vi "CameraControl.vi"() -> ()   [LabVIEW 2014]
uses:
  Libraries/atmcd32d.llb/ReadMode_mode typedef.ctl
  Libraries/atmcd32d.llb/AcquisitionMode_mode typedef.ctl
  Libraries/atmcd32d.llb/HSSpeed_type typedef.ctl
  Libraries/atmcd32d.llb/TriggerMode_mode typedef.ctl
  Libraries/atmcd32d.llb/Shutter_mode typedef.ctl
  Globals/AndorImage.vi
panel:
  in  "Take Video":bool
  out "Set Image Return":u32
  in  "Set Kinetic Series Number":i32=1
  in  "Set Number of Accumulations":i32=1
  in  "Set Horizontal Speed":u16(ring)=3 items=["1 MHz", "5 MHz", "10 MHz", "17 MHz"]
  out "Set Vertical Shift Speed Return":u32=20002
  in  "Set Vertical Shift Speed":u16(ring)=4 items=["0.3 us", "0.5 us", "0.9 us", "1.7 us", "3.3 us"]
  out "Vertical Shift Speed [us]":sgl format="%.1f"
  out "Set Shutter Return":u32=20002
  out "Intensity Graph":i32[][](graph)
  in  "vend":i32=512
  in  "vstart":i32=1
  in  "hend":i32=512
  in  "hstart":i32=1
  in  "vbin":i32=1
  in  "hbin":i32=1
  in  "Set Trigger":T1
  out "Return from Start Acquisition":u32=20002
  out "Return from Get Acquisition":u32=20002
  out "Exposure Time":sgl=0.01 format="%.2f"
  out "Return from GetStatus":u32=73
  in  "Take Image":bool=TRUE
  out "PreAmp Gains":i32=3
  out "EM Gain":u32
  out "Temperature [C]":i32=-70
  in  "Set EM Gain":i32
  in  "Read Settings":bool=TRUE
  in  "Stop":bool
  in  "Set Exposure Time [s]":sgl=0.01 format="%.2f"
  in  "Write Settings":bool
  in  "Set Temperature [C]":i32=-80
  out "DLL error code\n(20002 = Success)":u32=20002
  in  "Set Readout Amplifier":T2
  in  "Set Acquisition Mode":T3=enum."Kinetics"
  in  "Set Read Mode":T4=enum."Image"
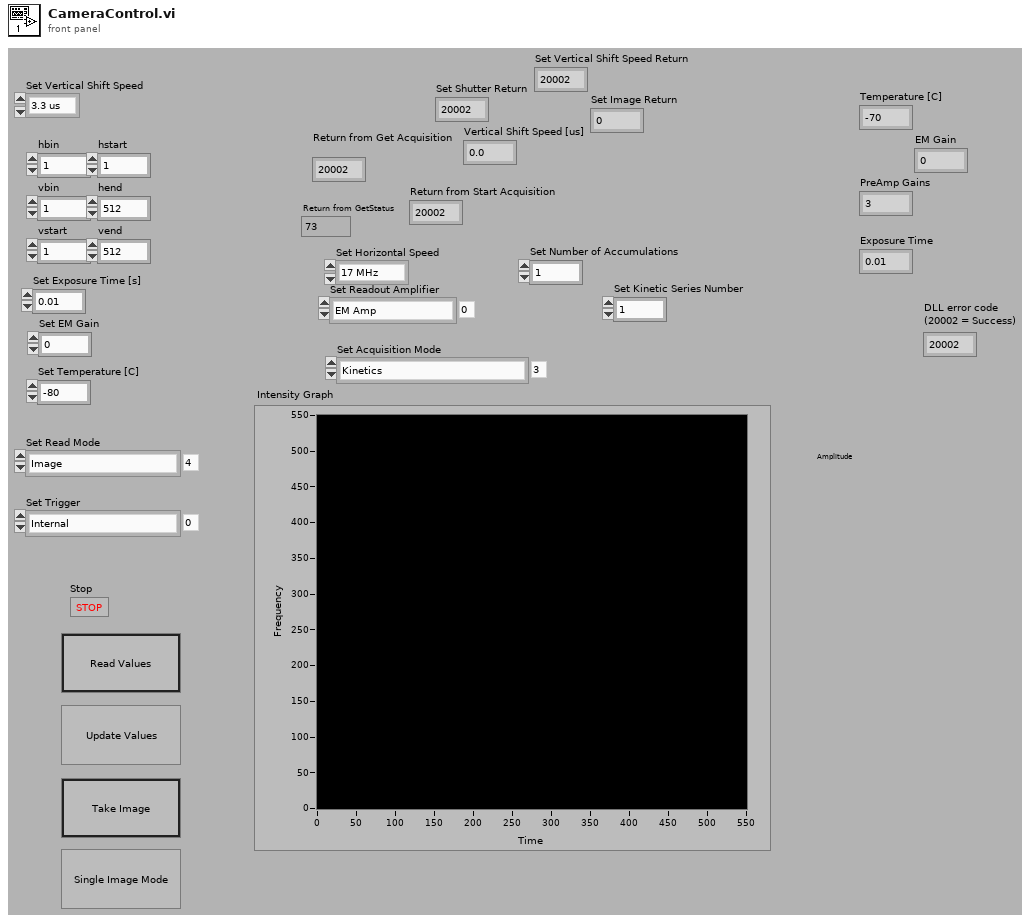
[diagram p1: front panel]
types:
  T1 = typedef "TriggerMode_mode typedef.ctl" = enum16{"Internal", "External", "N/A (2)", "N/A (3)", "N/A (4)", "N/A (5)", "External Start", "External Exposure (Bulb)", "N/A (8)", "External FVB EM", "Software", "N/A (11)", "External Charge Shifting"}
  T2 = typedef "HSSpeed_type typedef.ctl" = enum16{"EM Amp", "Conventional Amp"}
  T3 = typedef "AcquisitionMode_mode typedef.ctl" = enum16{"Reserved (0)", "Single Scan", "Accumulate", "Kinetics", "Fast Kinetics", "Run Till Abort", "Reserved (6)", "Reserved (7)", "Reserved (8)", "Time Delayed Integration"}
  T4 = typedef "ReadMode_mode typedef.ctl" = enum16{"Full Vertical Binning", "Multi-Track", "Random-Track", "Single-Track", "Image"}
  T5 = typedef "Shutter_mode typedef.ctl" = enum16{"Auto", "Open", "Close", "N/A (3)", "Open FVB Series", "Open Any Series"}
  T6 = typedef "Error Code Enum typedef.ctl" = enum32{"N/A (0)", "DRV_ERROR_CODES", "DRV_SUCCESS", "DRV_VXDNOTINSTALLED", "DRV_ERROR_SCAN", "DRV_ERROR_CHECK_SUM", "DRV_ERROR_FILELOAD", "DRV_UNKNOWN_FUNC", "DRV_ERROR_VXD_INIT", "DRV_ERROR_ADDRESS", "DRV_ERROR_PAGELOCK", "DRV_ERROR_PAGEUNLOCK", "DRV_ERROR_BOARDTEST", "DRV_ERROR_ACK", "DRV_ERROR_UP_FIFO", "DRV_ERROR_PATTERN", "N/A (16)", "DRV_ACQUISITION_ERRORS", "DRV_ACQ_BUFFER", "DRV_ACQ_DOWNFIFO_FULL", "DRV_PROC_UNKONWN_INSTRUCTION", "DRV_ILLEGAL_OP_CODE", "DRV_KINETIC_TIME_NOT_MET", "DRV_ACCUM_TIME_NOT_MET", "DRV_NO_NEW_DATA", "N/A (25)", "DRV_SPOOLERROR", "N/A (27)", "N/A (28)", "N/A (29)", "N/A (30)", "N/A (31)", "N/A (32)", "DRV_TEMPERATURE_CODES", "DRV_TEMPERATURE_OFF", "DRV_TEMPERATURE_NOT_STABILIZED", "DRV_TEMPERATURE_STABILIZED", "DRV_TEMPERATURE_NOT_REACHED", "DRV_TEMPERATURE_OUT_RANGE", "DRV_TEMPERATURE_NOT_SUPPORTED", "DRV_TEMPERATURE_DRIFT", "N/A (41)", "N/A (42)", "N/A (43)", "N/A (44)", "N/A (45)", "N/A (46)", "N/A (47)", "N/A (48)", "DRV_GENERAL_ERRORS", "DRV_INVALID_AUX", "DRV_COF_NOTLOADED", "DRV_FPGAPROG", "DRV_FLEXERROR", "DRV_GPIBERROR", "N/A (55)", "N/A (56)", "N/A (57)", "N/A (58)", "N/A (59)", "N/A (60)", "N/A (61)", "N/A (62)", "N/A (63)", "DRV_DATATYPE", "DRV_DRIVER_ERRORS", "DRV_P1INVALID", "DRV_P2INVALID", "DRV_P3INVALID", "DRV_P4INVALID", "DRV_INIERROR", "DRV_COFERROR", "DRV_ACQUIRING", "DRV_IDLE", "DRV_TEMPCYCLE", "DRV_NOT_INITIALIZED", "DRV_P5INVALID", "DRV_P6INVALID", "DRV_INVALID_MODE", "DRV_INVALID_FILTER", "DRV_I2CERRORS", "DRV_I2CDEVNOTFOUND", "DRV_I2CTIMEOUT", "DRV_P7INVALID", "N/A (84)", "N/A (85)", "N/A (86)", "N/A (87)", "N/A (88)", "N/A (89)", "DRV_IOCERROR", "DRV_VRMVERSIONERROR"}
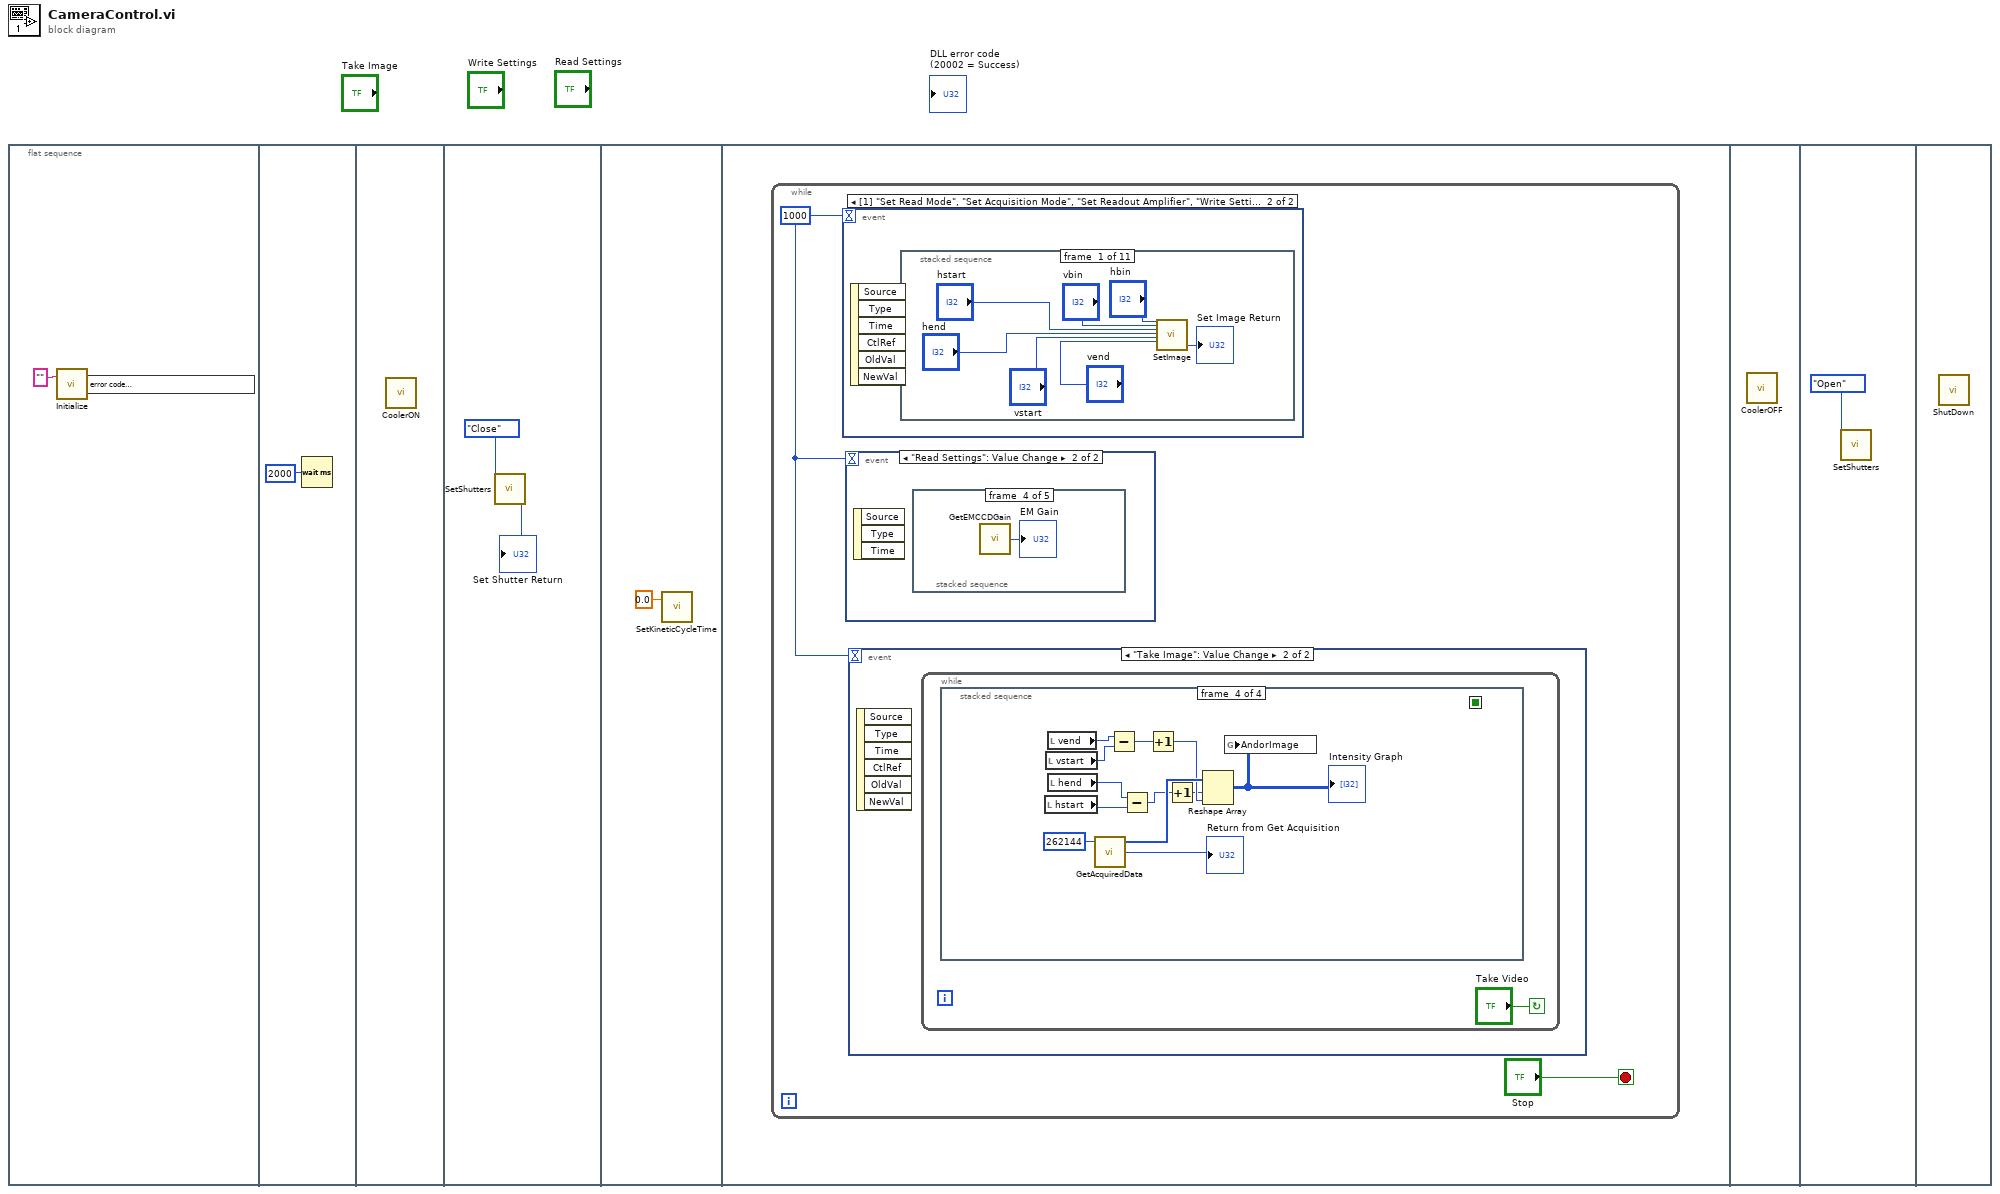
[diagram p0: block diagram]
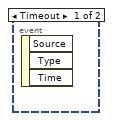
[diagram p2: hidden frame]
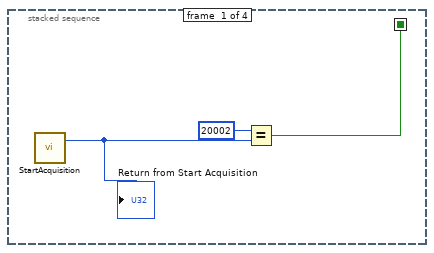
[diagram p3: hidden frame]
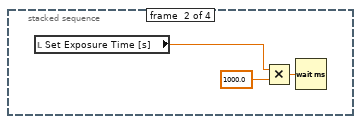
[diagram p4: hidden frame]
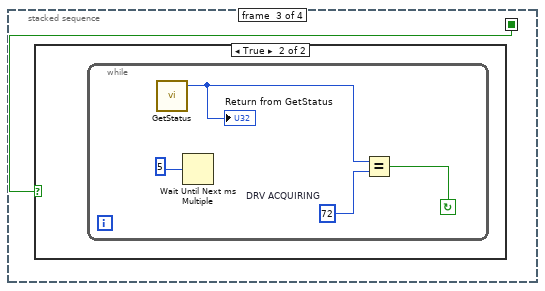
[diagram p5: hidden frame]
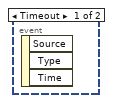
[diagram p7: hidden frame]
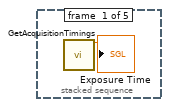
[diagram p8: hidden frame]
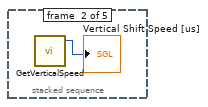
[diagram p9: hidden frame]
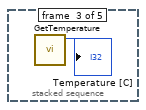
[diagram p10: hidden frame]
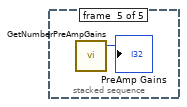
[diagram p11: hidden frame]
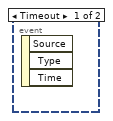
[diagram p12: hidden frame]
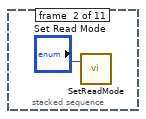
[diagram p13: hidden frame]
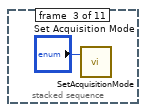
[diagram p14: hidden frame]
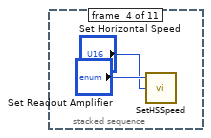
[diagram p15: hidden frame]
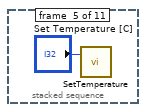
[diagram p16: hidden frame]
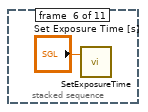
[diagram p17: hidden frame]
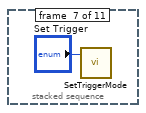
[diagram p18: hidden frame]
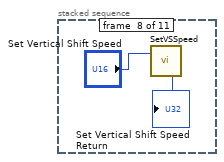
[diagram p19: hidden frame]
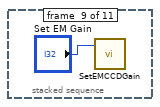
[diagram p20: hidden frame]
diagram:
  n1 = flat-sequence {
    frame #0 {
      n2 = call "Initialize.vi"("directory (\"\")"="" ("directory (\"\")")) -> ("DLL error code"=w1:u32)  [unwired: 1 in, 1 out]
      n3 = local write "DLL error code\n(20002 = Success)"(w1) -> ()
    }
    frame #1 {
      n4 = Wait (ms)(milliseconds to wait=u32 2000) -> ()  [unwired: 1 out]
    }
    frame #2 {
      n5 = call "CoolerON.vi"() -> ()  [unwired: 2 in, 2 out]
    }
    frame #3 {
      n6 = call "SetShutters.vi"("mode"=Shutter_mode_typedef."Close") -> ("DLL error code"=→"Set Shutter Return":u32)  [unwired: 17 in, 1 out]
    }
    frame #4 {
      n7 = call "SetKineticCycleTime.vi"("time"=sgl 0.0) -> ()  [unwired: 1 in, 2 out]
    }
    frame #5 {
      n8 = while {
        stop <- "Stop" stop-if-true
        w7 = 1000
        n9 = event shown="[1] \"Set Read Mode\", \"Set Acquisition Mode\", \"Set Readout Amplifier\", \"Write Settings\", \"Set Temperature [C]\", \"Set Exposure Time [s]\", \"Set Trigger\", \"hbin\", \"vbin\", \"hstart\", \"hend\", \"vstart\", \"vend\", \"Set EM Gain\", \"Set Vertical Shift Speed\", \"Set Vertical Shift Speed Return\", \"Set Horizontal Speed\", \"Set Number of Accumulations\", \"Set Kinetic Series Number\": Value Change" {
          selector: _ -> [_ _]
          dyn-events: _ -> [_ _]
          timeout: w7 -> [_ _]
          event Timeout {
            n10 = event-data() -> ()  [unwired: 1 in, 3 out]
          }
          event "Write Settings", "Set Temperature [C]", "Set Exposure Time [s]", "hbin", "vbin", "hstart", "hend", "vstart", "vend", "Set EM Gain", "Set Vertical Shift Speed", "Set Vertical Shift Speed Return", "Set Horizontal Speed", "Set Number of Accumulations", "Set Kinetic Series Number": Value Change {
            n11 = event-data() -> ()  [unwired: 1 in, 6 out]
            n12 = stacked-sequence {
              frame #0 {
                n13 = call "SetImage.vi"("hbin"="hbin", "vbin"="vbin", "hstart"="hstart", "hend"="hend", "vstart"="vstart", "vend"="vend") -> ("DLL error code"=→"Set Image Return":u32)  [unwired: 20 in, 1 out]
              }
              frame #1 {
                n14 = call "SetReadMode.vi"("mode"="Set Read Mode") -> ()  [unwired: 1 in, 2 out]
              }
              frame #2 {
                n15 = call "SetAcquisitionMode.vi"("mode"="Set Acquisition Mode") -> ()  [unwired: 1 in, 2 out]
              }
              frame #3 {
                n16 = call "SetHSSpeed.vi"("index"="Set Horizontal Speed", "type"="Set Readout Amplifier") -> ()  [unwired: 2 in, 2 out]
              }
              frame #4 {
                n17 = call "SetTemperature.vi"("temperature"="Set Temperature [C]") -> ()  [unwired: 1 in, 2 out]
              }
              frame #5 {
                n18 = call "SetExposureTime.vi"("time"="Set Exposure Time [s]") -> ()  [unwired: 1 in, 2 out]
              }
              frame #6 {
                n19 = call "SetTriggerMode.vi"("mode"="Set Trigger") -> ()  [unwired: 1 in, 2 out]
              }
              frame #7 {
                n20 = call "SetVSSpeed.vi"("index"="Set Vertical Shift Speed") -> ("DLL error code"=→"Set Vertical Shift Speed Return":u32)  [unwired: 1 in, 1 out]
              }
              frame #8 {
                n21 = call "SetEMCCDGain.vi"("gain"="Set EM Gain") -> ()  [unwired: 1 in, 2 out]
              }
              frame #9 {
                n22 = call "SetNumberAccumulations.vi"("number"="Set Number of Accumulations") -> ()  [unwired: 1 in, 2 out]
              }
              frame #10 {
                n23 = call "SetNumberKinetics.vi"("number"="Set Kinetic Series Number") -> ()  [unwired: 1 in, 2 out]
              }
            }
          }
        }
        n24 = event shown="[1] \"Read Settings\": Value Change" {
          selector: _ -> [_ _]
          dyn-events: _ -> [_ _]
          timeout: w7 -> [_ _]
          event Timeout {
            n25 = event-data() -> ()  [unwired: 1 in, 3 out]
          }
          event "Read Settings": Value Change {
            n26 = event-data() -> ()  [unwired: 1 in, 3 out]
            n27 = stacked-sequence {
              frame #0 {
                n28 = call "GetAcquisitionTimings.vi"() -> ("exposure"=→"Exposure Time":sgl)  [unwired: 11 in, 4 out]
              }
              frame #1 {
                n29 = call "GetVerticalSpeed.vi"() -> ("speed"=→"Vertical Shift Speed [us]":i32)  [unwired: 2 in, 2 out]
              }
              frame #2 {
                n30 = call "GetTemperature.vi"() -> ("temperature"=→"Temperature [C]":i32)  [unwired: 4 in, 3 out]
              }
              frame #3 {
                n31 = call "GetEMCCDGain.vi"() -> ("gain"=→"EM Gain":u32)  [unwired: 3 in, 2 out]
              }
              frame #4 {
                n32 = call "GetNumberPreAmpGains.vi"() -> ("number"=→"PreAmp Gains":i32)  [unwired: 3 in, 2 out]
              }
            }
          }
        }
        n33 = event shown="[1] \"Take Image\": Value Change" {
          selector: _ -> [_ _]
          dyn-events: _ -> [_ _]
          timeout: w7 -> [_ _]
          event Timeout {
            n34 = event-data() -> ()  [unwired: 1 in, 3 out]
          }
          event "Take Image": Value Change {
            n35 = event-data() -> ()  [unwired: 1 in, 6 out]
            n36 = while {
              stop <- "Take Video" continue-if-true
              n37 = stacked-sequence {
                seq-local: [w12 _ _ _] -> [_ _ w16 _]
                frame #0 {
                  n38 = call "StartAcquisition.vi"() -> ("DLL error code"=w11:u32)  [unwired: 2 in, 1 out]
                  "Return from Start Acquisition" <- w11
                  n39 = Equal?(x=u32 20002, y=w11) -> (x = y?=w12:bool)
                }
                frame #1 {
                  n40 = local read "Set Exposure Time [s]"() -> (w14:sgl)
                  n41 = Multiply(x=w14, y=sgl 1000.0) -> (x*y=w15:sgl)
                  n42 = Wait (ms)(milliseconds to wait=w15) -> ()  [unwired: 1 out]
                }
                frame #2 {
                  n43 = case shown="True" w16 {
                    frame False {
                    }
                    frame True {
                      n44 = while {
                        stop <- w19 continue-if-true
                        w18 = u16 72  # DRV ACQUIRING
                        n45 = call "GetStatus.vi"() -> ("status"=w17:T6)  [unwired: 3 in, 2 out]
                        "Return from GetStatus" <- w17
                        n46 = Wait Until Next ms Multiple(millisecond multiple=u32 5) -> ()  [unwired: 1 out]
                        n47 = Equal?(x=w17, y=w18) -> (x = y?=w19:bool)
                      }
                    }
                  }
                }
                frame #3 {
                  n48 = local read "hstart"() -> (w27:i32)
                  n49 = local read "vstart"() -> (w29:i32)
                  n50 = local read "vend"() -> (w30:i32)
                  n51 = local read "hend"() -> (w28:i32)
                  n52 = call "GetAcquiredData.vi"("size"=u32 262144) -> ("DLL error code"=→"Return from Get Acquisition":u32, "array"=w26:i32[])  [unwired: 2 in, 1 out]
                  n53 = Subtract(x=w30, y=w29) -> (x-y=w25:i32)
                  n54 = Subtract(x=w28, y=w27) -> (x-y=w24:i32)
                  n55 = Increment(x=w25) -> (x+1=w23:i32)
                  n56 = Increment(x=w24) -> (x+1=w22:i32)
                  n57 = Reshape Array(w26, w22, w23) -> (w21:i32[][])
                  "Intensity Graph" <- w21
                  n58 = global write "AndorImage.vi" "AndorImage"(w21) -> ()
                }
              }
            }
          }
        }
      }
    }
    frame #6 {
      n59 = call "CoolerOFF.vi"() -> ()  [unwired: 2 in, 2 out]
    }
    frame #7 {
      n60 = call "SetShutters.vi"("mode"=Shutter_mode_typedef."Open") -> ()  [unwired: 17 in, 2 out]
    }
    frame #8 {
      n61 = call "ShutDown.vi"() -> ()  [unwired: 2 in, 2 out]
    }
  }
